vi "TurnToAngleController.vi"(5 "MaxAccel":dbl, 7 "MaxVel":dbl, 8 "Reset":bool, 9 "Gains":T1={"FFV"=0.0032, "FFA"=0.0, "Vel PID"={"P"=0.0, "I"=0.0, "D"=0.0}} {"Vel PID"."D" format="%.3f"; "Vel PID"."I" format="%.3f"; "Vel PID"."P" format="%.3f"}, 10 "CurrentAngle":dbl, 11 "TargetAngle":dbl) -> (0 "Done":bool, 1 "Time Left":u32, 2 "RightPower":dbl, 3 "LeftPower":dbl, 4 "VelGraph":cluster{"Output":dbl, "dx/dt":dbl}(graph)={"Output"=47.4353047807108, "dx/dt"=76.52582126109495}, 6 "Pos":dbl(graph)=299.88802132939395)   [LabVIEW 2017]
panel:
  in  "StaticFrictionOvercomer":dbl=0.38 format="%#_13g"
  in  "Target Vel":dbl
  out "Power":dbl(graph)=299.88802132939395
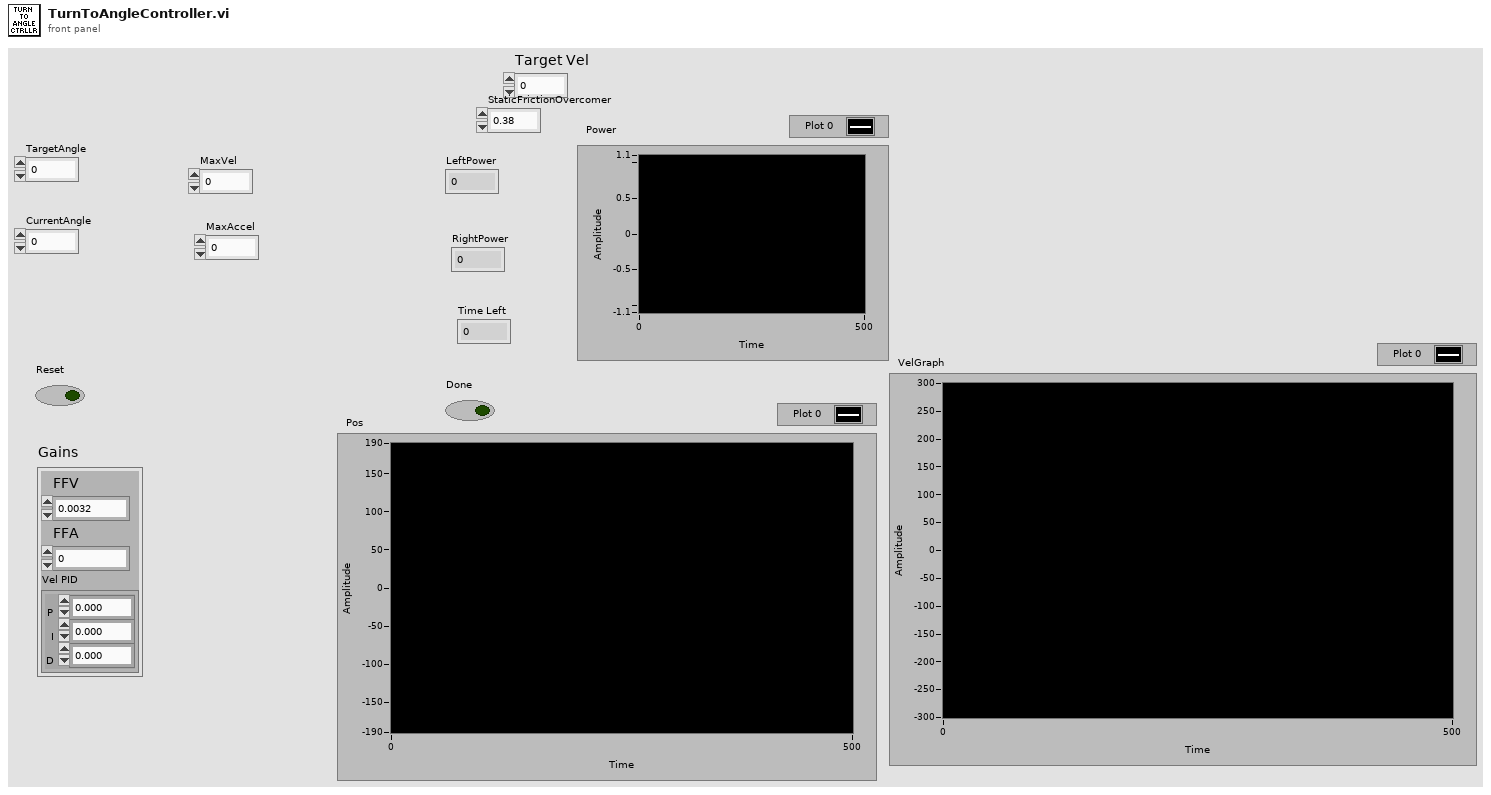
[diagram p1: front panel]
types:
  T1 = cluster{"FFV":dbl, "FFA":dbl, "Vel PID":cluster{"P":dbl, "I":dbl, "D":dbl}}
  T2 = cluster{"Profile":cluster{"Distances":dbl[], "Vels":dbl[]}, "CurrentAngle":dbl}
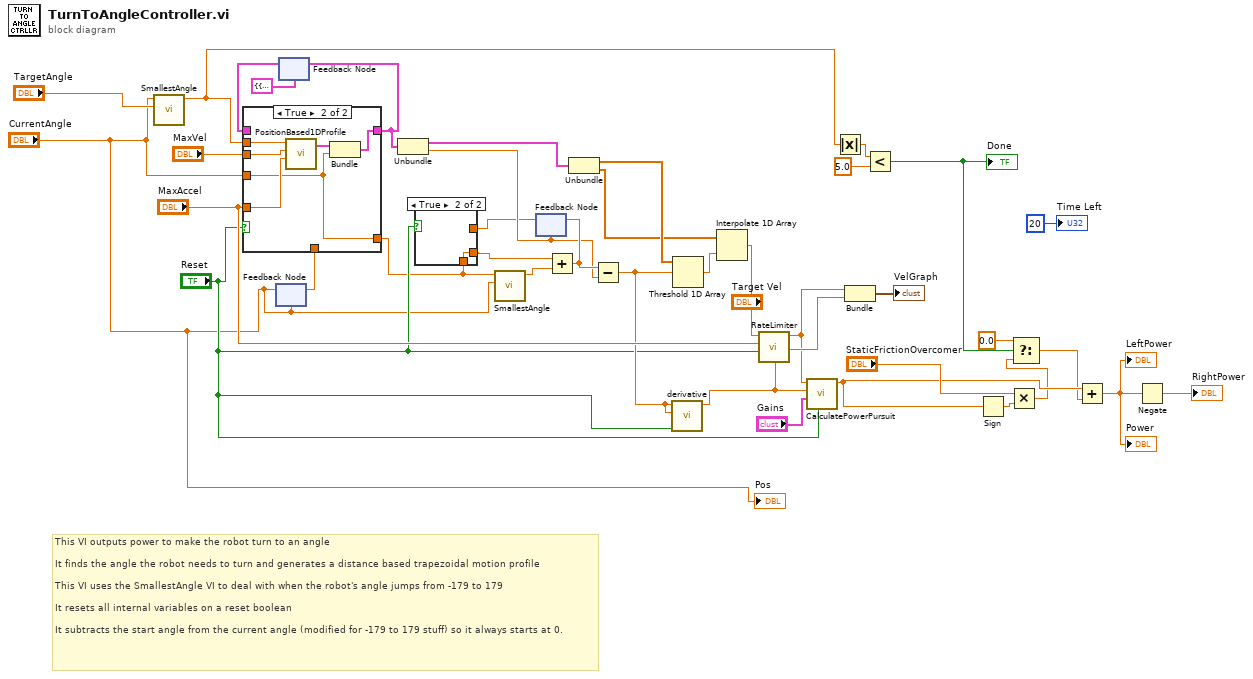
[diagram p0: block diagram]
diagram:
  # "This VI outputs power to make the robot turn to an angle\n\nIt finds the angle the robot needs to turn and generates a distance based trapezoidal motion profile\n\nThis VI uses the SmallestAngle VI to deal with when the robot's angle jumps from -179 to 179\n\nIt resets all internal variables on a reset boolean\n\nIt subtracts the start angle from the current angle (modified for -179 to 179 stuff) so it always starts at 0."
  n1 = call "SmallestAngle.vi"("Angle B"="TargetAngle", "Angle A"="CurrentAngle") -> ("Smallest A to B"=w20:dbl)  [unwired: 9 in]
  n2 = feedback #1("CurrentAngle") -> (w19:dbl)
  n3 = feedback-in #1("CurrentAngle") -> ()
  n4 = feedback #2(T2 {"Profile"={"Distances"=[], "Vels"=[]}, "CurrentAngle"=0.0}) -> (w36:T2)
  n5 = case shown="True" "Reset" {
    tunnel: w20 -> [_ w46]
    tunnel: "MaxVel" -> [_ w45]
    tunnel: "MaxAccel" -> [_ w44]
    tunnel: [w40 w43] -> w23
    tunnel: w36 -> [w40 _]
    tunnel: "CurrentAngle" -> [_ w41]
    tunnel: w19 -> [w39 _]
    tunnel: [w39 w41] -> w11
    frame False {
    }
    frame True {
      n6 = call "PositionBased1DProfile.vi"("MaxAccel"=w44, "MaxVel"=w45, "Distance"=w46) -> ("Profile"=w42:cluster{"Distances":dbl[], "Vels":dbl[]})  [unwired: 8 in]
      n7 = Bundle("Profile"=w42, "CurrentAngle"=w41) -> (w43:T2)  [unwired: 1 in]
    }
  }
  n8 = feedback-in #2(w23) -> ()
  n9 = Unbundle(w23) -> ("Profile"=w22:cluster{"Distances":dbl[], "Vels":dbl[]}, "CurrentAngle"=w17:dbl)
  n10 = call "SmallestAngle.vi"("Angle B"="CurrentAngle", "Angle A"=w11) -> ("Smallest A to B"=w21:dbl)  [unwired: 9 in]
  n11 = feedback #3(w17) -> (w13:dbl)
  n12 = case shown="True" "Reset" {
    tunnel: [w47 w48] -> w14
    tunnel: w13 -> [w47 _]
    tunnel: w11 -> [_ w48]
    frame False {
    }
    frame True {
    }
  }
  n13 = Add(x=w14, y=w21) -> (x+y=w18:dbl)
  n14 = feedback-in #3(w18) -> ()
  n15 = Unbundle(w22) -> ("Distances"=w35:dbl[], "Vels"=w34:dbl[])
  n16 = Subtract(x=w18, y=w17) -> (x-y=w15:dbl)
  n17 = call "derivative.vi"("Reset"="Reset", "Starting value"=w15, "x"=w15) -> ("dx/dt"=w16:dbl)  [unwired: 8 in]
  n18 = Threshold 1D Array(2:w15, 3:w35) -> (0:w33:dbl)  [unwired: 1 in]
  n19 = Interpolate 1D Array(1:w33, 2:w34) -> (0:w32:dbl)
  n20 = call "RateLimiter.vi"("Reset"="Reset", "Max dx/dt"="MaxAccel", "Input"=w32) -> ("Output"=w9:dbl)  [unwired: 8 in]
  n21 = call "CalculatePowerPursuit.vi"("Reset"="Reset", "Gains"="Gains", "Vel"=w16, "Target Vel"=w9) -> ("Power"=w6:dbl)  [unwired: 7 in]
  n22 = Absolute Value(x=w20) -> (abs(x)=w29:dbl)
  n23 = Bundle("Output"=w9, "dx/dt"=w16) -> (→"VelGraph":cluster{"Output":dbl, "dx/dt":dbl})  [unwired: 1 in]
  n24 = Less?(x=w29, y=5.0) -> (x < y?=w5:bool)
  "Done" <- w5
  n25 = Sign(1:w6) -> (0:w8:dbl)
  n26 = Multiply(x="StaticFrictionOvercomer", y=w8) -> (x*y=w3:dbl)
  n27 = Select(t=0.0, s=w5, f=w3) -> (s? t:f=w2:dbl)
  n28 = Add(x=w6, y=w2) -> (x+y=w1:dbl)
  "LeftPower" <- w1
  "Power" <- w1
  n29 = Negate(x=w1) -> (-x=→"RightPower":dbl)
  "Time Left" <- u32 20 ("Time Left")
  "Pos" <- "CurrentAngle"
